vi "AO Continuous FPGA.vi"() -> ()   [LabVIEW 2019]
uses:
  <vilib>/rvi/Emulation/niFpgaGetClockAttributes.vi
  <vilib>/rvi/Emulation/niFpgaSctlEmulationGetInTimedLoop.vi
  <vilib>/rvi/Emulation/niFpgaEmulationReportErrorSimple.vi
  <vilib>/rvi/interface/RandomDataEmulation/nirviRandomDataMultiElementFPGAFIFO.vi
  <instcachedir>/0/nirviRandomDataMultiElementFPGAFIFO_1ED88BA00AC641F388A9B1FAA20E354D.lvgen/nirviRandomDataMultiElementFPGAFIFO_1ED88BA00AC641F388A9B1FAA20E354D_005.vi
  <vilib>/rvi/interface/RandomDataEmulation/niFpgaRandomDataHandleErrors.vi
  <vilib>/rvi/Emulation/niFpgaCriticalErrorInLSC.vi
  <vilib>/rvi/Emulation/niFpgaEmulationIsFPGAContextNoSignature.vi
  <vilib>/rvi/errors/niFpgaSetErrorForExecOnDevCompSimple.vi
  <vilib>/rvi/eio/common/nirviEmuReportErrorAndStop.vi
  <vilib>/rvi/DataTransferAndStorage/Container/Common/niFpgaContainerGetUniqueNameForEmu.vi
  <vilib>/rvi/FIFO/Fifo_Resource/nirvififoEmulationSetSize.vi
  <vilib>/rvi/FIFO/Fifo_Resource/nirviFifoEmulationQueueMgr.vi
  <instcachedir>/0/nirviFifoEmulationQueueMgr_E5CAEC123FF24DC58D834DCA3CDAA9B5.lvgen/nirviFifoEmulationQueueMgr_E5CAEC123FF24DC58D834DCA3CDAA9B5_004.vi
  <vilib>/rvi/FIFO/Fifo_Resource/nirvififoEmulationDetermineInputValidOut.vi
  <vilib>/rvi/FIFO/Fifo_Resource/nirvififoEmulationCreateLock.vi
  <vilib>/rvi/Emulation/niFpgaProcessEmulError.vi
  <vilib>/rvi/FIFO/Fifo_Resource/nirvififoEmulationObtainLock.vi
  <vilib>/rvi/FIFO/Fifo_Resource/nirvififoEmulationReleaseLock.vi
  <vilib>/rvi/occurrence/nirviWaitOnOccurrenceBase.vi
  <vilib>/rvi/errors/nirviReportUnexpectedCaseInternalError.vi
  <vilib>/rvi/errors/nirviReportUnexpectedCaseInternalError (U32).vi
  <vilib>/Utility/error.llb/Clear Errors.vi
  <vilib>/rvi/eio/common/nirviEmuTemplateMethod_errors.vi
  <vilib>/rvi/DataTransferAndStorage/Container/Common/niFpgaContainerSetEmuInfo.vi
  <vilib>/rvi/DataTransferAndStorage/Container/XNode/niFpgaContainer.xnode
  <vilib>/rvi/interface/RandomDataEmulation/nirviRandomDataFpgaMultiElementTemplate.vi
  <vilib>/rvi/FIFO/Fifo_Resource/nirvififoEmulationWrite.vi
  <vilib>/rvi/FIFO/Fifo_Resource/nirvififoEmulationRead.vi
  <vilib>/eio/EIONode/EIONode.xnode
  <vilib>/rvi/LocalResourceManager/LocalResourceManager.xnode
panel:
  in  "开始":bool
  in  "B1.Enable":bool
  in  "B0.Enable":bool
  in  "A1.Enable":bool
  in  "A0.Enable":bool
  in  "CNTR":u32=200
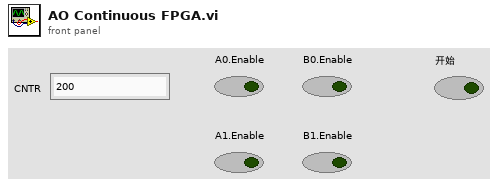
[diagram p1: front panel]
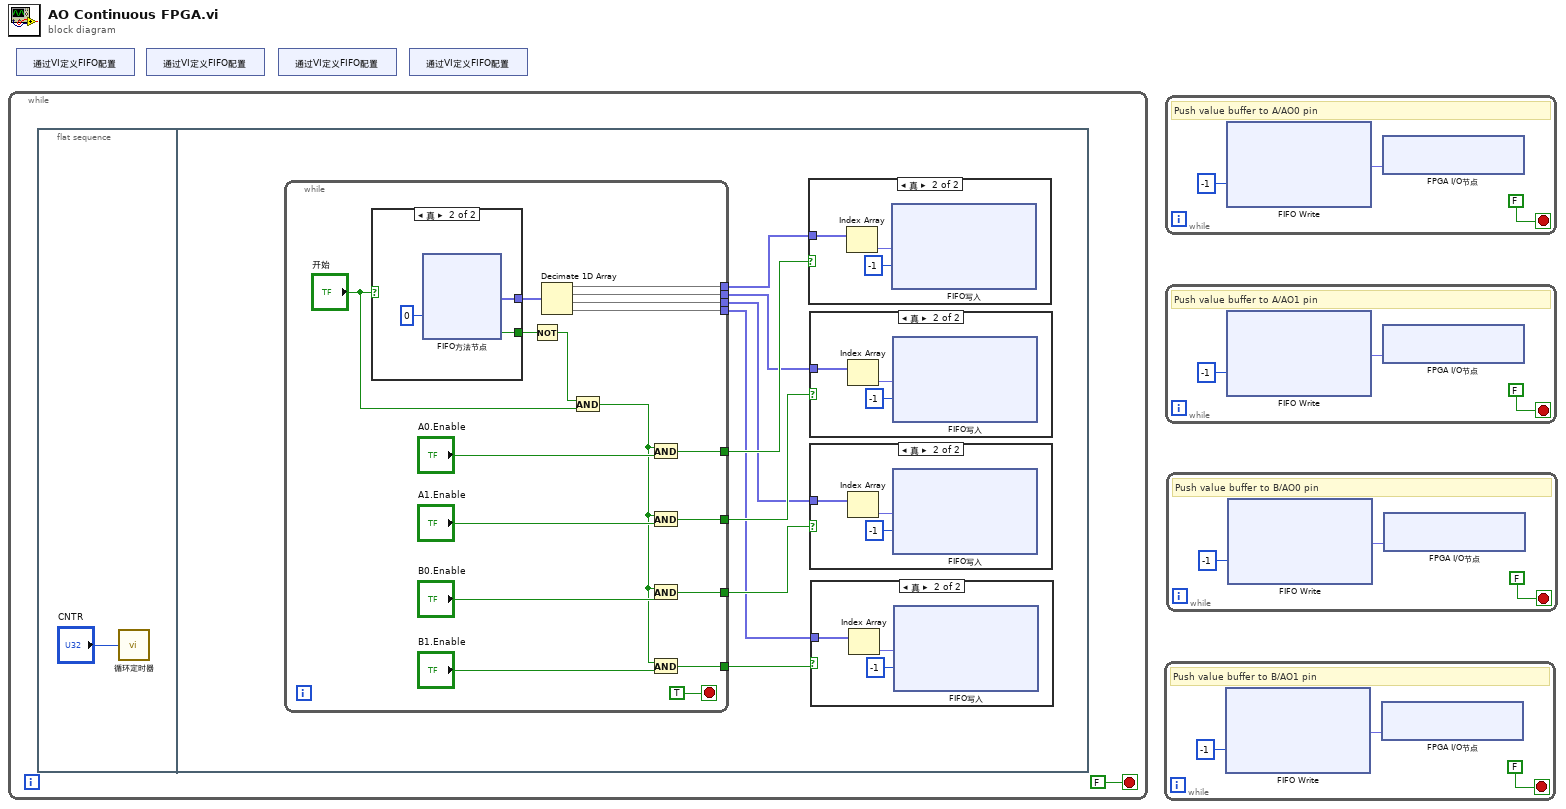
[diagram p0: block diagram]
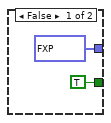
[diagram p2: hidden frame]
diagram:
  n1 = while {
    stop <- FALSE stop-if-true
    n2 = flat-sequence {
      frame #0 {
        n3 = call "循环定时器"("Count(Ticks)"="CNTR") -> ()  [unwired: 1 out]
      }
      frame #1 {
        n4 = while {
          tunnel: [w20] -> w10
          tunnel: [w19] -> w5
          tunnel: [w18] -> w4
          tunnel: [w17] -> w3
          tunnel: [w16] -> w9
          tunnel: [w15] -> w6
          tunnel: [w14] -> w7
          tunnel: [w13] -> w8
          stop <- TRUE stop-if-true
          n5 = case shown="真" "开始" {
            tunnel: [TRUE ("超时？") w32] -> w28
            tunnel: [fxp<+/-,20,5>[] [0.0, 0.0, 0.0, 0.0] ("元素") w31] -> w11
            frame False {
            }
            frame True {
              n6 = xnode ("FIFO方法节点")("超时"=0) -> ("元素"=w31:fxp<+/-,20,5>[], "超时？"=w32:bool)  [unwired: 1 in, 1 out]
            }
          }
          n7 = Not(x=w28) -> (.not. x?=w27:bool)
          n8 = Decimate 1D Array(w11) -> (w20:fxp<+/-,20,5>[], w19:fxp<+/-,20,5>[], w18:fxp<+/-,20,5>[], w17:fxp<+/-,20,5>[])
          n9 = And(x=w27, y="开始") -> (x .and. y?=w21:bool)
          n10 = And(x=w21, y="A0.Enable") -> (x .and. y?=w16:bool)
          n11 = And(x=w21, y="A1.Enable") -> (x .and. y?=w15:bool)
          n12 = And(x=w21, y="B0.Enable") -> (x .and. y?=w14:bool)
          n13 = And(x=w21, y="B1.Enable") -> (x .and. y?=w13:bool)
        }
        n14 = case shown="真" w9 {
          tunnel: w10 -> [_ w45]
          frame False {
          }
          frame True {
            n15 = Index Array(array=w45) -> (element=w44:fxp<+/-,20,5>)  [unwired: 1 in]
            n16 = xnode ("FIFO写入")("元素"=w44, "超时"=-1) -> ()  [unwired: 1 in, 2 out]
          }
        }
        n17 = case shown="真" w6 {
          tunnel: w5 -> [_ w42]
          frame False {
          }
          frame True {
            n18 = Index Array(array=w42) -> (element=w41:fxp<+/-,20,5>)  [unwired: 1 in]
            n19 = xnode ("FIFO写入")("元素"=w41, "超时"=-1) -> ()  [unwired: 1 in, 2 out]
          }
        }
        n20 = case shown="真" w7 {
          tunnel: w4 -> [_ w39]
          frame False {
          }
          frame True {
            n21 = Index Array(array=w39) -> (element=w38:fxp<+/-,20,5>)  [unwired: 1 in]
            n22 = xnode ("FIFO写入")("元素"=w38, "超时"=-1) -> ()  [unwired: 1 in, 2 out]
          }
        }
        n23 = case shown="真" w8 {
          tunnel: w3 -> [_ w36]
          frame False {
          }
          frame True {
            n24 = Index Array(array=w36) -> (element=w35:fxp<+/-,20,5>)  [unwired: 1 in]
            n25 = xnode ("FIFO写入")("元素"=w35, "超时"=-1) -> ()  [unwired: 1 in, 2 out]
          }
        }
      }
    }
  }
  n26 = xnode "通过VI定义FIFO配置"() -> ()  [unwired: 1 out]
  n27 = xnode "通过VI定义FIFO配置"() -> ()  [unwired: 1 out]
  n28 = xnode "通过VI定义FIFO配置"() -> ()  [unwired: 1 out]
  n29 = xnode "通过VI定义FIFO配置"() -> ()  [unwired: 1 out]
  n30 = while {
    stop <- FALSE stop-if-true
    # "Push value buffer to B/AO1 pin"
    n31 = xnode ("FIFO Write")("超时"=-1 ("Timeout")) -> ("元素"=w47:fxp<+/-,20,5>)  [unwired: 1 in, 2 out]
    n32 = xnode "FPGA I/O节点"("ConnectorB/AO1"=w47) -> ()  [unwired: 1 in, 1 out]
  }
  n33 = while {
    stop <- FALSE stop-if-true
    # "Push value buffer to A/AO0 pin"
    n34 = xnode ("FIFO Write")("超时"=-1 ("Timeout")) -> ("元素"=w50:fxp<+/-,20,5>)  [unwired: 1 in, 2 out]
    n35 = xnode "FPGA I/O节点"("ConnectorA/AO0"=w50) -> ()  [unwired: 1 in, 1 out]
  }
  n36 = while {
    stop <- FALSE stop-if-true
    # "Push value buffer to A/AO1 pin"
    n37 = xnode ("FIFO Write")("超时"=-1 ("Timeout")) -> ("元素"=w53:fxp<+/-,20,5>)  [unwired: 1 in, 2 out]
    n38 = xnode "FPGA I/O节点"("ConnectorA/AO1"=w53) -> ()  [unwired: 1 in, 1 out]
  }
  n39 = while {
    stop <- FALSE stop-if-true
    # "Push value buffer to B/AO0 pin"
    n40 = xnode ("FIFO Write")("超时"=-1 ("Timeout")) -> ("元素"=w56:fxp<+/-,20,5>)  [unwired: 1 in, 2 out]
    n41 = xnode "FPGA I/O节点"("ConnectorB/AO0"=w56) -> ()  [unwired: 1 in, 1 out]
  }
